vi "Get_Di_Array.vi"(0 "reference in":refnum<class "FPGA_Concrete.lvclass">, 11 "error in (no error)":errorcluster) -> (4 "reference out":refnum<class "FPGA_Concrete.lvclass">, 6 "DIs":bool[](array[boolean]), 15 "error out":errorcluster)   [LabVIEW 2019, in "FPGA_Concrete.lvclass"]
uses:
  FPGA_Concrete.lvclass
  FPGA_Concrete.lvclass/FPGA_Concrete.ctl
  <vilib>/Utility/error.llb/Error Cluster From Error Code.vi
  <vilib>/rvi/errors/niLvFpgaAdjustHostInterfaceError.vi
  <vilib>/rvi/interface/nirviReadWriteControl/nirviReadWriteControl.xnode
  FPGA VI Reference.ctl
  NiFpgaLv.dll
  <vilib>/rvi/interface/Simulation/niFpgaSimulationCallBeginRW.vi
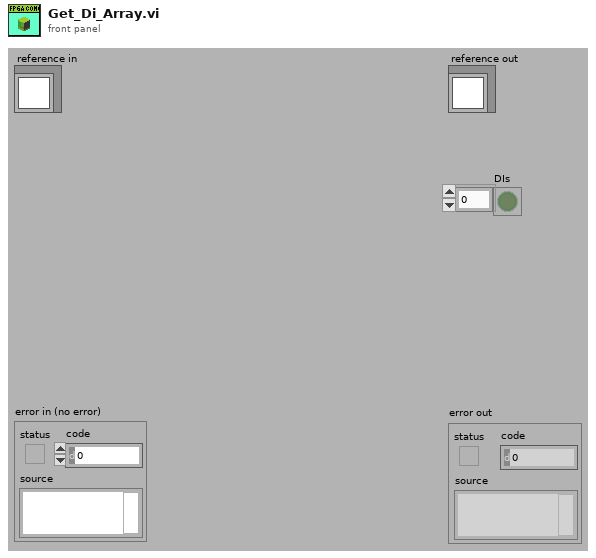
[diagram p1: front panel]
types:
  T1 = typedef "FPGA_Concrete.lvclass/FPGA VI Reference.ctl" = refnum<k20>
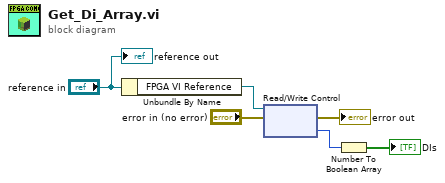
[diagram p0: block diagram]
diagram:
  n1 = Unbundle By Name("reference in") -> ("FPGA VI Reference"=w5:T1)
  n2 = xnode "Read/Write Control"("FPGA VI Reference In"=w5, "error in"="error in (no error)") -> ("error out"=→"error out":errorcluster, "DIs"=w2:u32)  [unwired: 1 out]
  n3 = Number To Boolean Array(number=w2) -> (Boolean array=→"DIs":bool[])
  "reference out" <- "reference in"
